vi "Save Settings.vi"(1 "This VI":refnum<vi>, 2 "Path":path, 3 "Array":bool[](array[boolean])) -> ()   [LabVIEW 2023]
panel:
  out "Class Name":string
  out "Class ID":u32
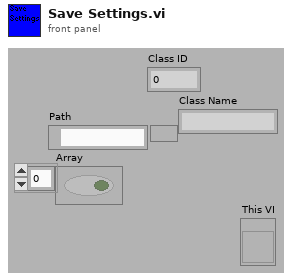
[diagram p1: front panel]
types:
  T1 = enum16{"open", "replace", "create", "open or create", "replace or create", "replace or create with confirmation"}
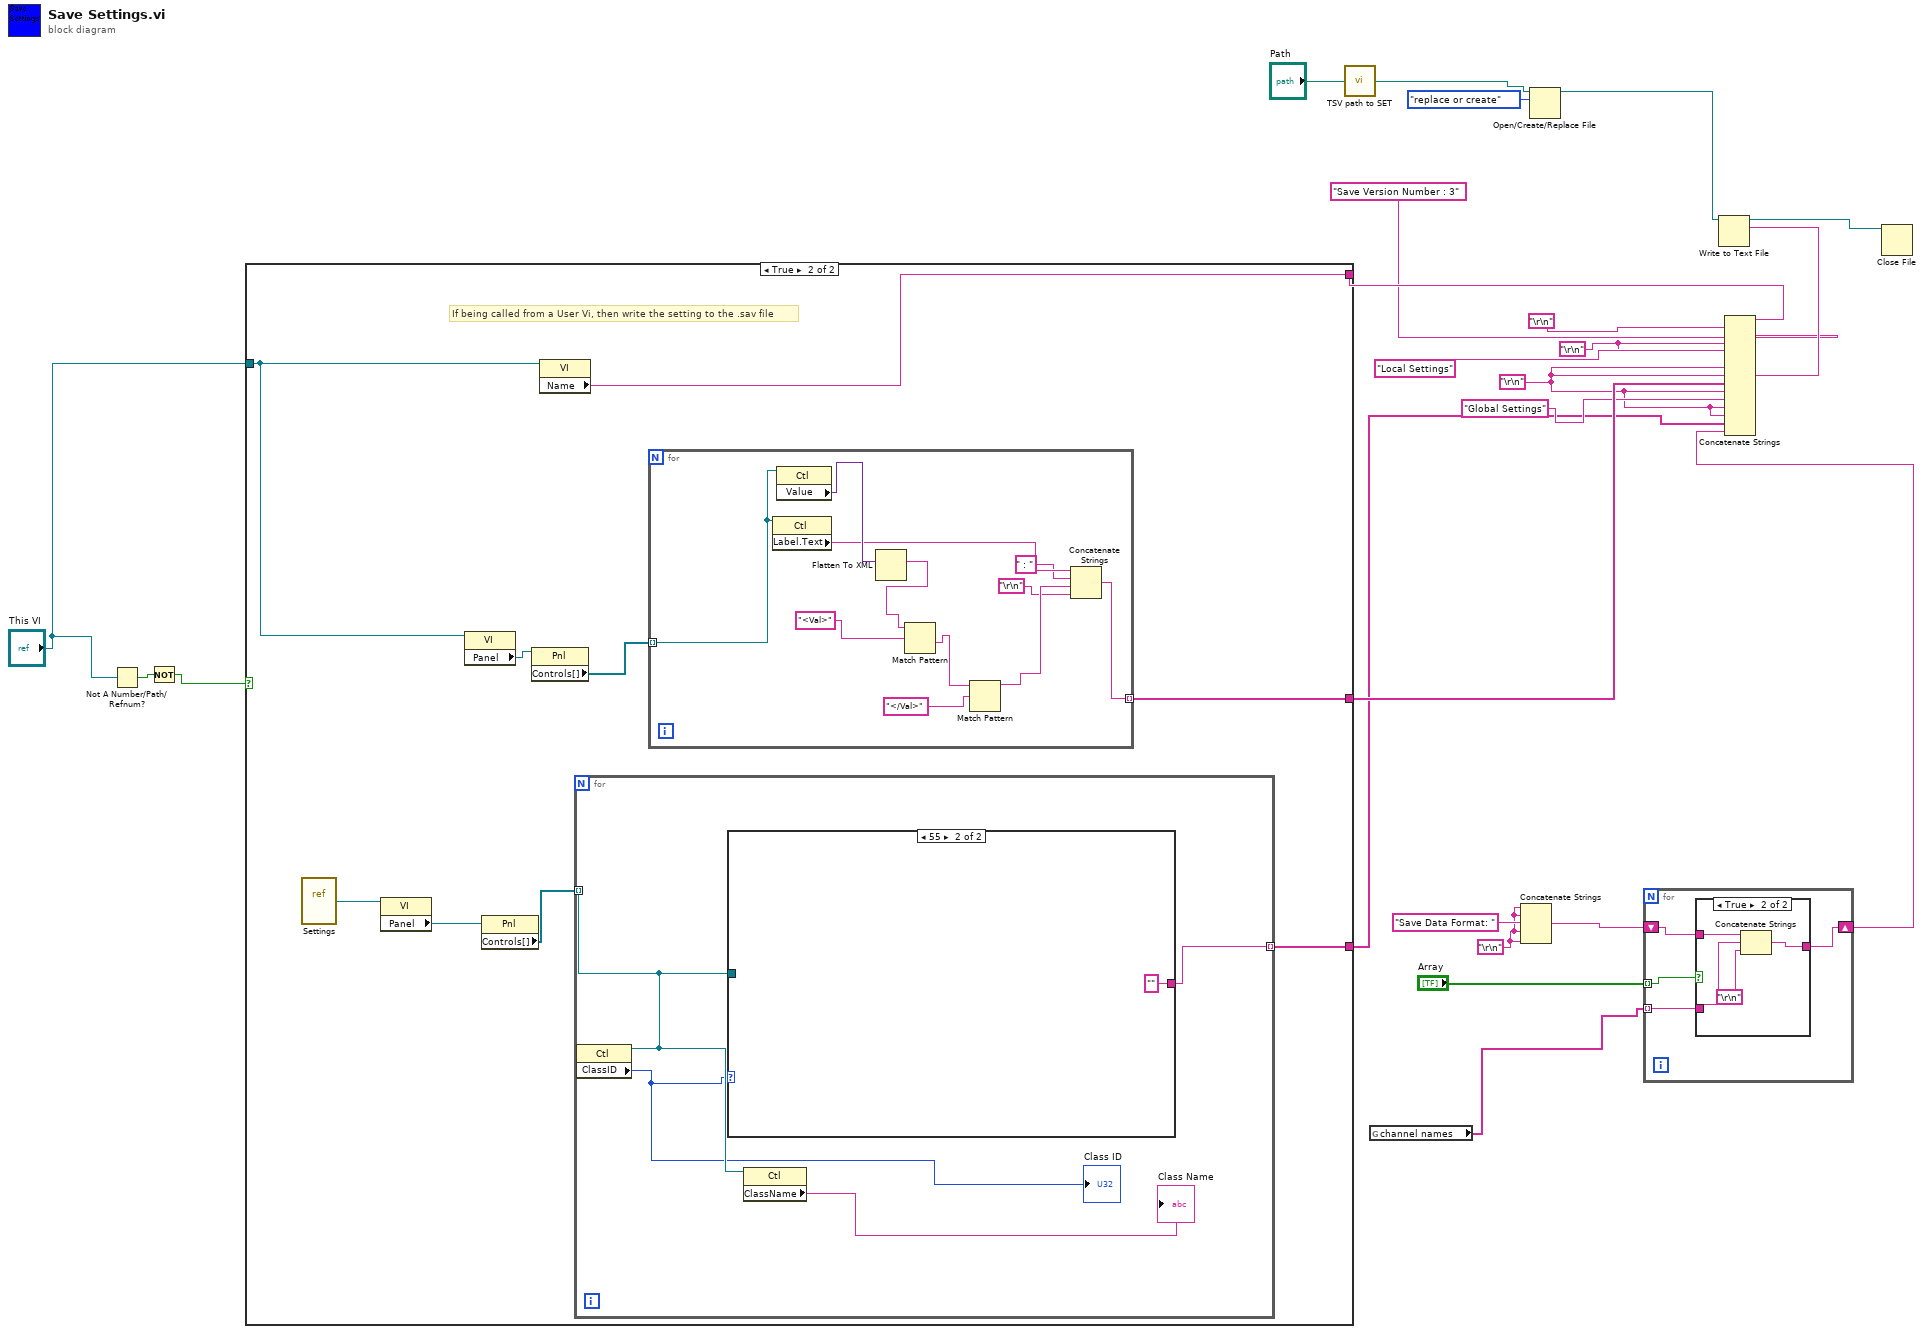
[diagram p0: block diagram]
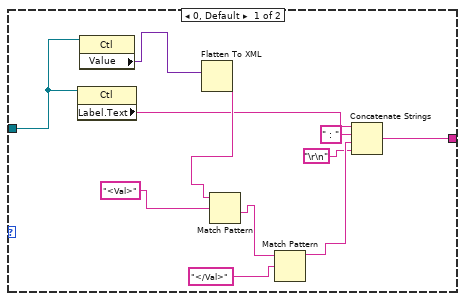
[diagram p3: hidden frame]
diagram:
  w3 = "\r\n"
  w18 = "\r\n"
  w4 = "\r\n"
  n1 = Not A Number/Path/Refnum?(number/path/refnum="This VI") -> (NaN/Path/Refnum?=w14:bool)
  n2 = Not(x=w14) -> (.not. x?=w11:bool)
  n3 = case shown="True" w11 {
    tunnel: [_ w33] -> w22
    tunnel: [_ w25] -> w5
    tunnel: [_ w29] -> w19
    tunnel: "This VI" -> [_ w26]
    frame False {
    }
    frame True {
      # "If being called from a User Vi, then write the setting to the .sav file"
      n4 = vi-ref "Settings.vi"() -> (w30:refnum<vi>)
      n5 = property class="VI"(reference=w30) -> ("Panel"=w32:refnum<vi>)  [unwired: 1 in, 2 out]
      n6 = property class="VI"(reference=w26) -> ("Panel"=w27:refnum<vi>)  [unwired: 1 in, 2 out]
      n7 = property class="Pnl"(reference=w32) -> ("Controls[]"=w31:refnum<vi>[])  [unwired: 1 in, 2 out]
      n8 = property class="Pnl"(reference=w27) -> ("Controls[]"=w28:refnum<vi>[])  [unwired: 1 in, 2 out]
      n9 = property class="VI"(reference=w26) -> ("Name"=w29:string)  [unwired: 1 in, 2 out]
      n10 = for {
        tunnel: w31 -> [w47] mode=indexing
        tunnel: [w48] -> w25 mode=indexing
        n11 = property class="Ctl"(reference=w47) -> ("ClassID"=w45:u32)  [unwired: 1 in, 2 out]
        "Class ID" <- w45
        n12 = case shown="55" w45 {
          tunnel: [w51 ""] -> w48
          tunnel: w47 -> [w49 _]
          frame 0, Default {
            n13 = property class="Ctl"(reference=w49) -> ("Label.Text"=w54:string)  [unwired: 1 in, 2 out]
            n14 = property class="Ctl"(reference=w49) -> ("Value"=w59:variant)  [unwired: 1 in, 2 out]
            n15 = Flatten To XML(6:w59) -> (2:w58:string)
            n16 = Match Pattern(string=w58, regular expression="<Val>") -> (after substring=w56:string)  [unwired: 1 in, 3 out]
            n17 = Match Pattern(string=w56, regular expression="</Val>") -> (before substring=w53:string)  [unwired: 1 in, 3 out]
            n18 = Concatenate Strings(w54, " : " ("string"), w53, "\r\n") -> (w51:string)
          }
          frame 55 {
          }
        }
        n19 = property class="Ctl"(reference=w47) -> ("ClassName"=→"Class Name":string)  [unwired: 1 in, 2 out]
      }
      n20 = for {
        tunnel: w28 -> [w34] mode=indexing
        tunnel: [w36] -> w33 mode=indexing
        n21 = property class="Ctl"(reference=w34) -> ("Label.Text"=w39:string)  [unwired: 1 in, 2 out]
        n22 = property class="Ctl"(reference=w34) -> ("Value"=w44:variant)  [unwired: 1 in, 2 out]
        n23 = Flatten To XML(6:w44) -> (2:w43:string)
        n24 = Match Pattern(string=w43, regular expression="<Val>") -> (after substring=w41:string)  [unwired: 1 in, 3 out]
        n25 = Match Pattern(string=w41, regular expression="</Val>") -> (before substring=w38:string)  [unwired: 1 in, 3 out]
        n26 = Concatenate Strings(w39, " : " ("string"), w38, "\r\n") -> (w36:string)
      }
    }
  }
  n27 = call "TSV path to SET.vi"("*.tsv path"="Path") -> ("*.set path"=w10:path)
  n28 = global read "Settings.vi" "channel names"() -> (w1:string[])
  n29 = Concatenate Strings(w3, w3, "Save Data Format: ", w3, w3) -> (w16:string)
  n30 = Open/Create/Replace File(file path (use dialog)=w10, operation (0:open)=T1."replace or create") -> (refnum out=w9:refnum<file>)  [unwired: 4 in, 2 out]
  n31 = for {
    tunnel: w1 -> [w61] mode=indexing
    shift-right: [w63] -> w6
    shift-left: w16 -> [w64]
    tunnel: "Array" -> [w62] mode=indexing
    n32 = case shown="True" w62 {
      tunnel: w64 -> [w65 w69]
      tunnel: [w65 w68] -> w63
      tunnel: w61 -> [_ w67]
      frame False {
      }
      frame True {
        n33 = Concatenate Strings(w69, w67, "\r\n") -> (w68:string)
      }
    }
  }
  n34 = Concatenate Strings(w19, "\r\n", "Save Version Number : 3" ("string"), w18, w18, "Local Settings", w4, w4, w22, w4, "Global Settings", w4, w4, w5, w6) -> (w23:string)
  n35 = Write to Text File(file (use dialog)=w9, text=w23) -> (refnum out=w8:refnum<file>)  [unwired: 1 in, 3 out]
  n36 = Close File(refnum=w8) -> ()  [unwired: 1 in, 2 out]
